vi "test.workspace_create_datasource_and_connection_without_specifying_workspace.vi"   [LabVIEW 2020]
uses:
  730c9c5b-7bb2-47cf-818b-6e2ed47344d4.vi
  Nominal Client/Nominal Client.lvclass
  <vilib>/addons/_JKI Toolkits/Caraya/classes/Test/Test.lvclass
  <vilib>/addons/_JKI Toolkits/Caraya/classes/Assert/Assert.lvclass
  <vilib>/addons/_JKI Toolkits/Caraya/classes/Assert/Assert Error.vi
  <vilib>/addons/_JKI Toolkits/Caraya/classes/Assert/Assert Not Error.vi
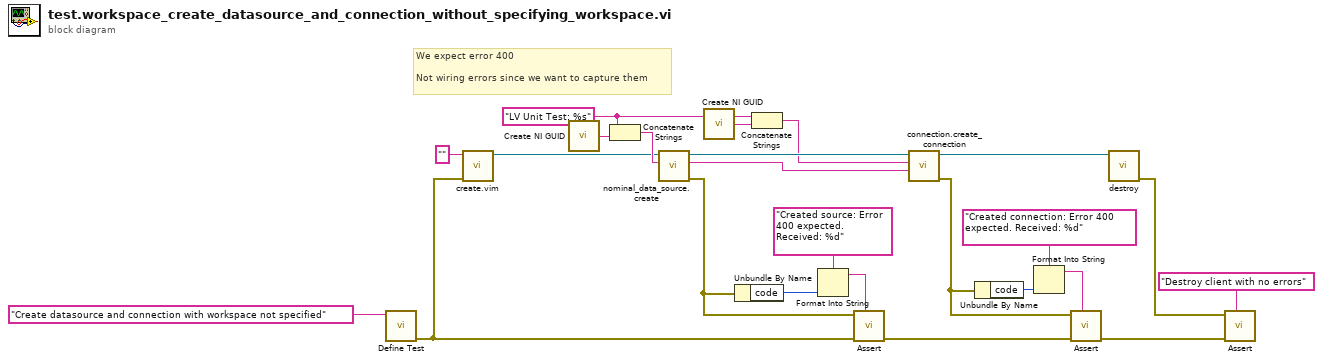
[diagram p0: block diagram]
diagram:
  w11 = "LV Unit Test: %s" ("format string")
  # "We expect error 400\n\nNot wiring errors since we want to capture them"
  n1 = call <vilib>:"Define Test.vi"("Label (VI Title)"="Create datasource and connection with workspace not specified") -> ("error out"=w9:errorcluster)  [unwired: 9 in, 1 out]
  n2 = call "create.vim"("error in"=w9, "API Token (string or path)"="" ("Workspace RID (string or path)")) -> ("Nominal Client"=w10:refnum<class "Nominal Client.lvclass">)  [unwired: 8 in, 1 out]
  n3 = call <vilib>:"Create NI GUID.vi"() -> ("NI GUID"=w12:string)
  n4 = Concatenate Strings(w11, w12) -> (w18:string)
  n5 = call "nominal_data_source.create.vi"("Name"=w18, "Nominal Client in"=w10) -> ("error out"=w8:errorcluster, "rid"=w16:string, "Nominal Client out"=w17:refnum<class "Nominal Client.lvclass">)  [unwired: 6 in, 1 out]
  n6 = call <vilib>:"Create NI GUID.vi"() -> ("NI GUID"=w13:string)
  n7 = Unbundle By Name(w8) -> ("code"=w6:i32)
  n8 = Concatenate Strings(w11, w13) -> (w15:string)
  n9 = Format Into String(format string="Created source: Error 400 expected. Received: %d" ("Label"), w6) -> (resulting string=w5:string)  [unwired: 2 in, 1 out]
  n10 = call-poly <vilib>:"Assert.vi"("Label"=w5, "error in (no error)"=w9, "Error?"=w8) -> ("error out"=w14:errorcluster)  [unwired: 7 in, 1 out]
  n11 = call "connection.create_connection.vi"("nominalDataSourceRid"=w16, "name"=w15, "Nominal Client in"=w17) -> ("error out"=w1:errorcluster, "Nominal Client out"=w20:refnum<class "Nominal Client.lvclass">)  [unwired: 5 in, 2 out]
  n12 = Unbundle By Name(w1) -> ("code"=w2:i32)
  n13 = Format Into String(format string="Created connection: Error 400 expected. Received: %d" ("Label"), w2) -> (resulting string=w3:string)  [unwired: 2 in, 1 out]
  n14 = call-poly <vilib>:"Assert.vi"("Label"=w3, "error in (no error)"=w14, "Error?"=w1) -> ("error out"=w19:errorcluster)  [unwired: 7 in, 1 out]
  n15 = call "destroy.vi"("Nominal Client"=w20) -> ("error out"=w22:errorcluster)  [unwired: 10 in]
  n16 = call-poly <vilib>:"Assert.vi"("Label"="Destroy client with no errors", "error in (no error)"=w19, "Not Error?"=w22) -> ()  [unwired: 7 in, 2 out]
